vi "Server Cluster.vi"() -> (0 "Cluster":T1)   [LabVIEW 2011]
doc: "Cluster for the Server in the QDMH Client-Server demonstration.\n\nAAL 9/09"
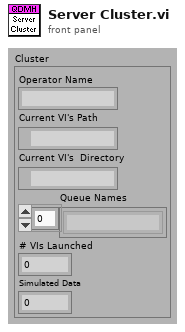
[diagram p1: front panel]
types:
  T1 = cluster{"Operator Name":string, "Current VI's Path":path, "Current VI's  Directory":path, "Queue Names":string[], "# VIs Launched":i32, "Simulated Data":dbl}
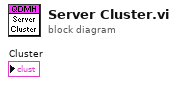
[diagram p0: block diagram]
diagram:
